vi "WriteInJournalProc.vi"(8 "error in (no error)":errorcluster, 10 "InstrumentEnum":T1, 11 "Event":string) -> (0 "error out":errorcluster)   [LabVIEW 2017]
doc: "Use this template to build a VI to use as a subVI."
uses:
  IntrumentEnum.ctl
  SpectroMeasurementCtrlEnum.ctl
  Database/DatabaseContollerGFVenum.ctl
  JournalCluster.ctl
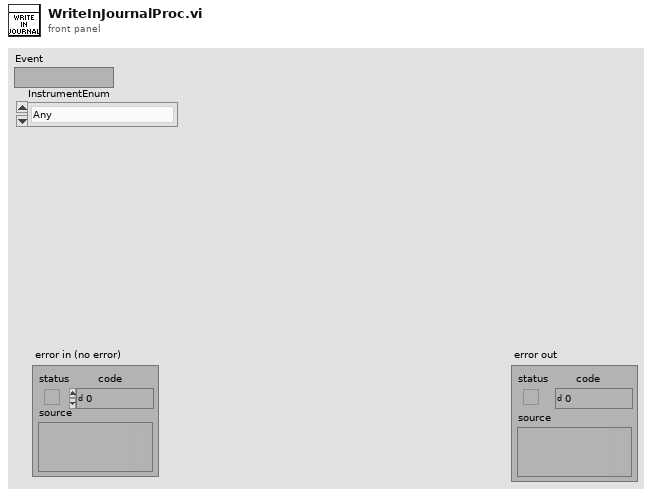
[diagram p1: front panel]
types:
  T1 = typedef "IntrumentEnum.ctl" = enum16{"Any", "RamanSpectrometer", "Microscope", "Stage"}
  T2 = typedef "DatabaseContollerGFVenum.ctl" = enum16{"Init and Open Database!", "Get next Journal Number!", "WriteInJournalTable", "GetNewMeas_dataIndex", "UpdateWithSpectrometerData", "UpdateWithMicroscopeData", "UpdateWithMapScriptData", "UpdateWithmainUIData", "Get Objective Microns/Pixels", "Get User Name!", "Get Active Users Names!", "Get User Picture!", "Get User Phone Number!", "Get Setup Names!", "Get Active Microscope Objectives!", "Get Experiment Number!", "Get Sample Types!", "Write meas_conf Table", "Write meas_data Table", "GetListOfIndices", "Get Objective Index"}
  T3 = typedef "JournalCluster.ctl" = cluster{"idJournal":u32, "Event Time Stamp":timestamp, "Event":string, "idUsers":u32, "idmeas_setup":u32, "idmeas_script":u32, "InstrumentEnum":T1}
  T4 = typedef "SpectroMeasurementCtrlEnum.ctl" = enum16{"Init", "InsertMeasurementScript", "InsertSetupIndex", "InsertCurrentUserIndex", "GetAllData!"}
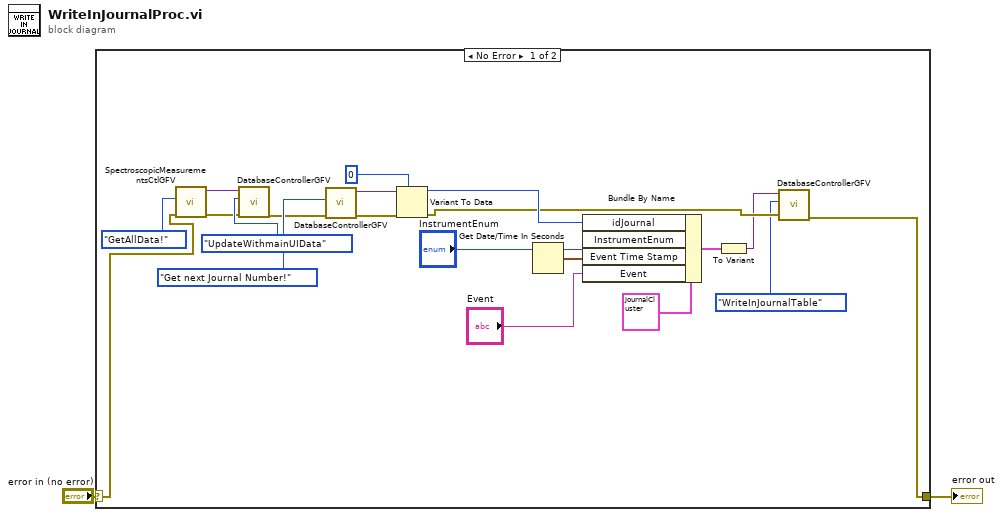
[diagram p0: block diagram]
diagram:
  n1 = case shown="No Error" "error in (no error)" {
    selector: "error in (no error)" -> [w6 w23]
    tunnel: [w5 w23] -> w1
    frame No Error {
      n2 = call "SpectroscopicMeasurementsCtlGFV.vi"("error in (no error)"=w6, "Enum"=SpectroMeasurementCtrlEnum."GetAllData!") -> ("error out"=w19:errorcluster, "Data Out"=w21:variant)  [unwired: 8 in]
      n3 = call "DatabaseControllerGFV.vi"("error in (no error)"=w19, "Enum"=DatabaseContollerGFVenum."UpdateWithmainUIData", "Data in"=w21) -> ("error out"=w14:errorcluster)  [unwired: 7 in, 1 out]
      n4 = call "DatabaseControllerGFV.vi"("error in (no error)"=w14, "Enum"=DatabaseContollerGFVenum."Get next Journal Number!") -> ("error out"=w15:errorcluster, "Data Out"=w13:variant)  [unwired: 8 in]
      n5 = Variant To Data(error in=w15, type=0, Variant=w13) -> (data=w11:i32, error out=w10:errorcluster)
      n6 = Get Date/Time In Seconds() -> (seconds since 1Jan1904=w17:timestamp)
      n7 = Bundle By Name(cluster=T3 {"idJournal"=0, "Event Time Stamp"=timestamp(0 s since 1904-01-01), "Event"="", "idUsers"=0, "idmeas_setup"=0, "idmeas_script"=0, "InstrumentEnum"=enum."Stage"}, "idJournal"=w11, "InstrumentEnum"="InstrumentEnum", "Event Time Stamp"=w17, "Event"="Event") -> (w9:T3)
      n8 = To Variant(anything=w9) -> (Variant=w8:variant)
      n9 = call "DatabaseControllerGFV.vi"("error in (no error)"=w10, "Enum"=DatabaseContollerGFVenum."WriteInJournalTable", "Data in"=w8) -> ("error out"=w5:errorcluster)  [unwired: 7 in, 1 out]
    }
    frame Error {
    }
  }
  "error out" <- w1
